vi "Set Name XML.vi"(1 "Name XML File":string, 2 "Synapses in":refnum<class "Synapses.lvclass">) -> (0 "Synapses out":refnum<class "Synapses.lvclass">)   [LabVIEW 2013, in "Synapses.lvclass"]
uses:
  Synapses.lvclass
  Synapses.lvclass/Synapses.ctl
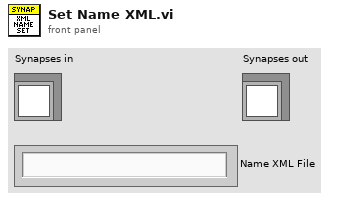
[diagram p1: front panel]
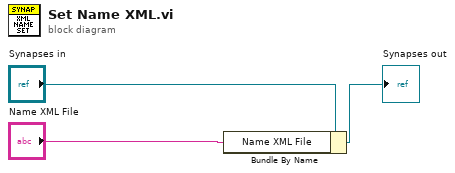
[diagram p0: block diagram]
diagram:
  n1 = Bundle By Name(cluster="Synapses in", "Name XML File"="Name XML File") -> (→"Synapses out":refnum<class "Synapses.lvclass">)
